vi "IBM4_Diff_Read(I1).vi"(8 "error in":errorcluster, 9 "Neg-Chan":enum16{"A2", "A3", "A4", "A5"}(ring)=enum."A3", 10 "Pos-Chan":enum16{"A2", "A3", "A4", "A5"}(ring), 11 "COM resource in":refnum<visa-resource-name>="COM9") -> (0 "error out":errorcluster, 2 "output":i32, 3 "COM resource out":refnum<visa-resource-name>)   [LabVIEW 2021, in "IBM4.lvlib"]
doc: "This VI interfaces with the IBM4 to perform a differential read operation.\n\nThe output will in binary format (thus, integer).\nOnly a single read operation is made with this VI. \n\nAlternate read operations exist covering binary or floating point, single reading, multiple readings, and an average of multiple readings (floating point only)."
uses:
  <instrlib>/IBM4/IBM4.lvlib
panel:
  out "error out 2":errorcluster
  out "read buffer":string
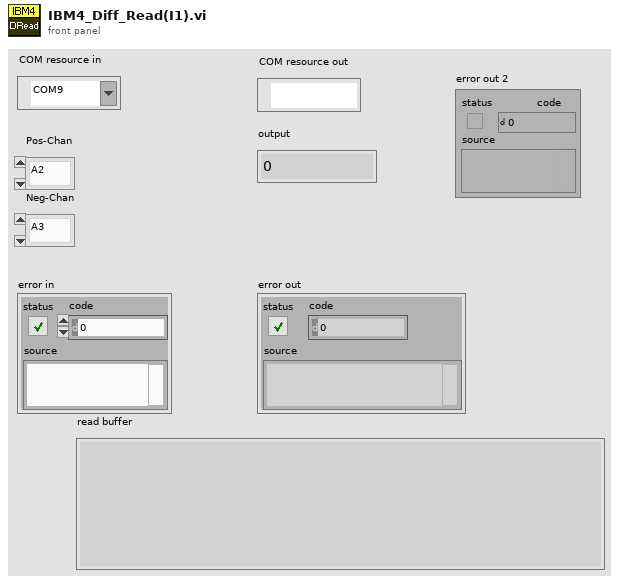
[diagram p1: front panel]
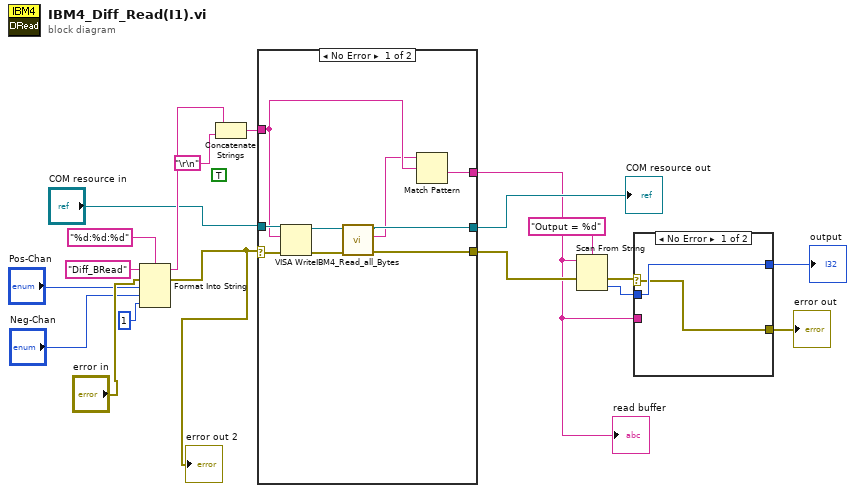
[diagram p0: block diagram]
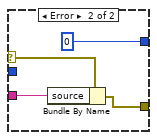
[diagram p2: hidden frame]
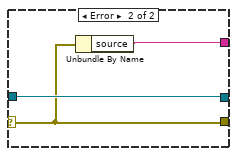
[diagram p3: hidden frame]
diagram:
  (unwired) TRUE ("Enable Termination\nChar (T)")
  n1 = Format Into String(format string="%d:%d:%d", initial string="Diff_BRead", error in="error in", "Pos-Chan", "Neg-Chan", 1 ("input 2")) -> (resulting string=w12:string, error out=w3:errorcluster)
  "error out 2" <- w3
  n2 = Concatenate Strings(w12, "\r\n") -> (w11:string)
  n3 = case shown="No Error" w3 {
    selector: w3 -> [w25 w29]
    tunnel: "COM resource in" -> [w28 w31]
    tunnel: [w21 w29] -> w15
    tunnel: [w27 w30] -> w7
    tunnel: w11 -> [w26 _]
    tunnel: [w22 w31] -> w16
    frame No Error {
      n4 = VISA Write(VISA resource name=w28, write buffer=w26, error in (no error)=w25) -> (VISA resource name out=w24:refnum<visa-resource-name>, error out=w23:errorcluster)  [unwired: 1 out]
      n5 = call <instrlib>:"IBM4_Read_all_Bytes.vi"("error in (no error)"=w23, "VISA Refnum in"=w24) -> ("error out"=w21:errorcluster, "String"=w20:string, "VISA Refnum out"=w22:refnum<visa-resource-name>)  [unwired: 3 in]
      n6 = Match Pattern(string=w20, regular expression=w26) -> (after substring=w27:string)  [unwired: 1 in, 3 out]
    }
    frame Error {
      n7 = Unbundle By Name(w29) -> ("source"=w30:string)
    }
  }
  "COM resource out" <- w16
  "read buffer" <- w7
  n8 = Scan From String(format string="Output = %d", input string=w7, error in=w15) -> (error out=w10:errorcluster, output 1=w5:i32)  [unwired: 2 in, 2 out]
  n9 = case shown="No Error" w10 {
    selector: w10 -> [w32 w36]
    tunnel: w5 -> [w33 _]
    tunnel: [w33 0] -> w9
    tunnel: [w32 w34] -> w8
    tunnel: w7 -> [_ w35]
    frame No Error {
    }
    frame Error {
      n10 = Bundle By Name(cluster=w36, "source"=w35) -> (w34:errorcluster)
    }
  }
  "error out" <- w8
  "output" <- w9
